vi "EINDE2.vi"() -> ()   [LabVIEW 2018]
uses:
  Kleuren- en afstandsensor/FSM States.ctl
  FSM States Project TOTAAL.ctl
panel:
  out "Initial State":T1=enum."MOVE DOWNWARDS"
  out "Tussentijd":i32
  out "Timer":i32
  out "The End":bool
  in  "stop 3":bool
  in  "ON/OFF Grijper":bool
  in  "stop":bool
  in  "Aantal Witte blokjes":dbl
  in  "Aantal rode blokjes":dbl
  in  "Aantal Zwarte blokjes":dbl
  in  "LED aansturen":bool[](array[boolean])
  out "Current State":T1
  out "Motor":bool[](array[boolean])
  out "State to recover from":T1=enum."Stilstaan"
  in  "EMERGENCY":bool
  in  "Teller wit":dbl
  in  "Teller Rood":dbl
  in  "Teller zwart":dbl
  out "Wit":bool
  out "Zwart":bool
  out "Rood":bool
  in  "Kleurmaken":bool
  out "Kleuren veranderen":T2
  out "Analoge in":dbl[](array[numeric]) format="%0.2f"
  out "Afstand":bool
  # "INPUT"
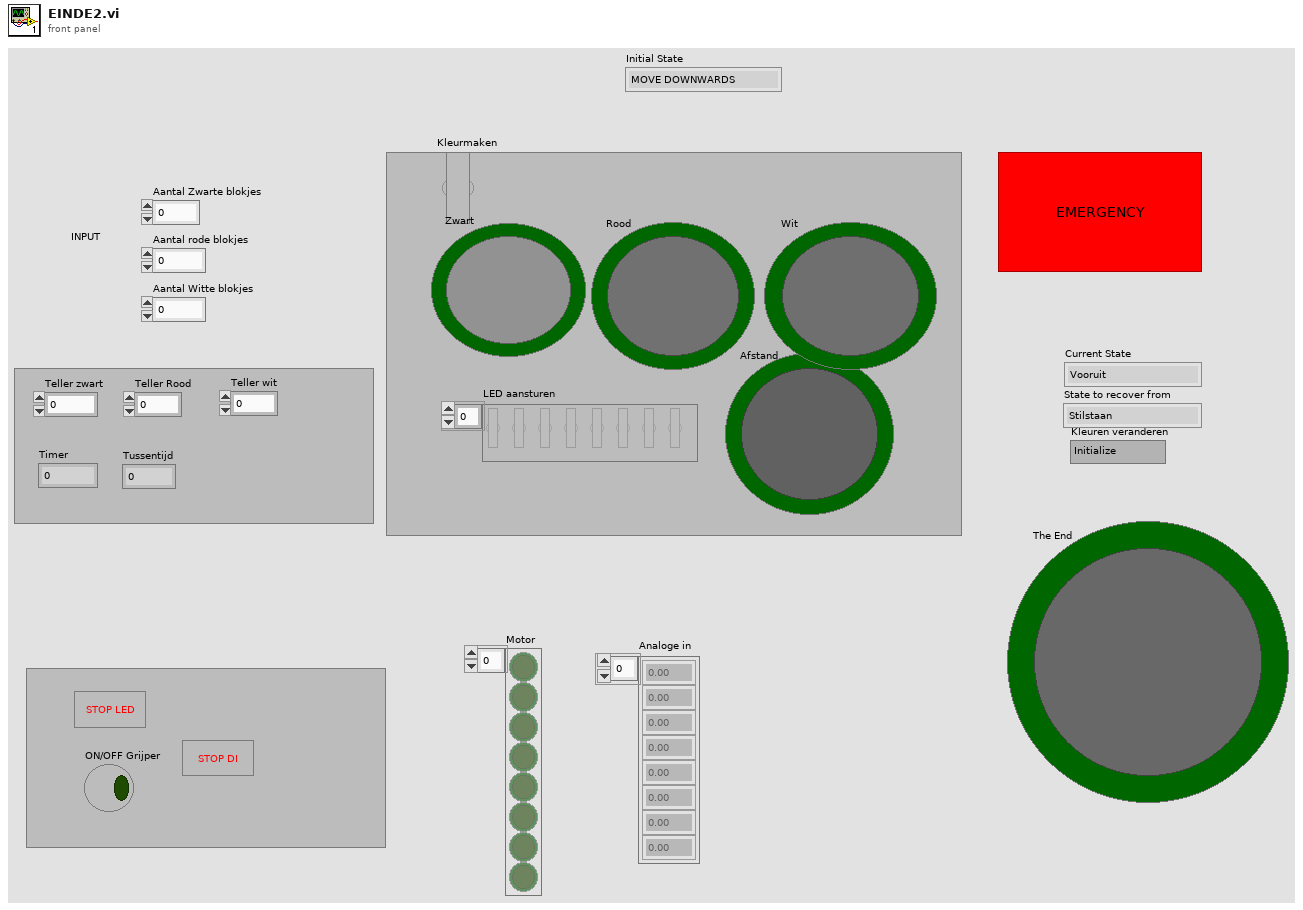
[diagram p1: front panel]
types:
  T1 = typedef "FSM States Project TOTAAL.ctl" = enum16{"Vooruit", "Achteruit", "Stilstaan", "EMERGENCY", "MOVE DOWNWARDS", "GRAB", "MOVE UPWARDS", "ROTATE", "DROP", "RETURN", "Stop "}
  T2 = typedef "FSM States.ctl" = enum16{"Initialize", "ROOD", "GROEN ", "Blauw "}
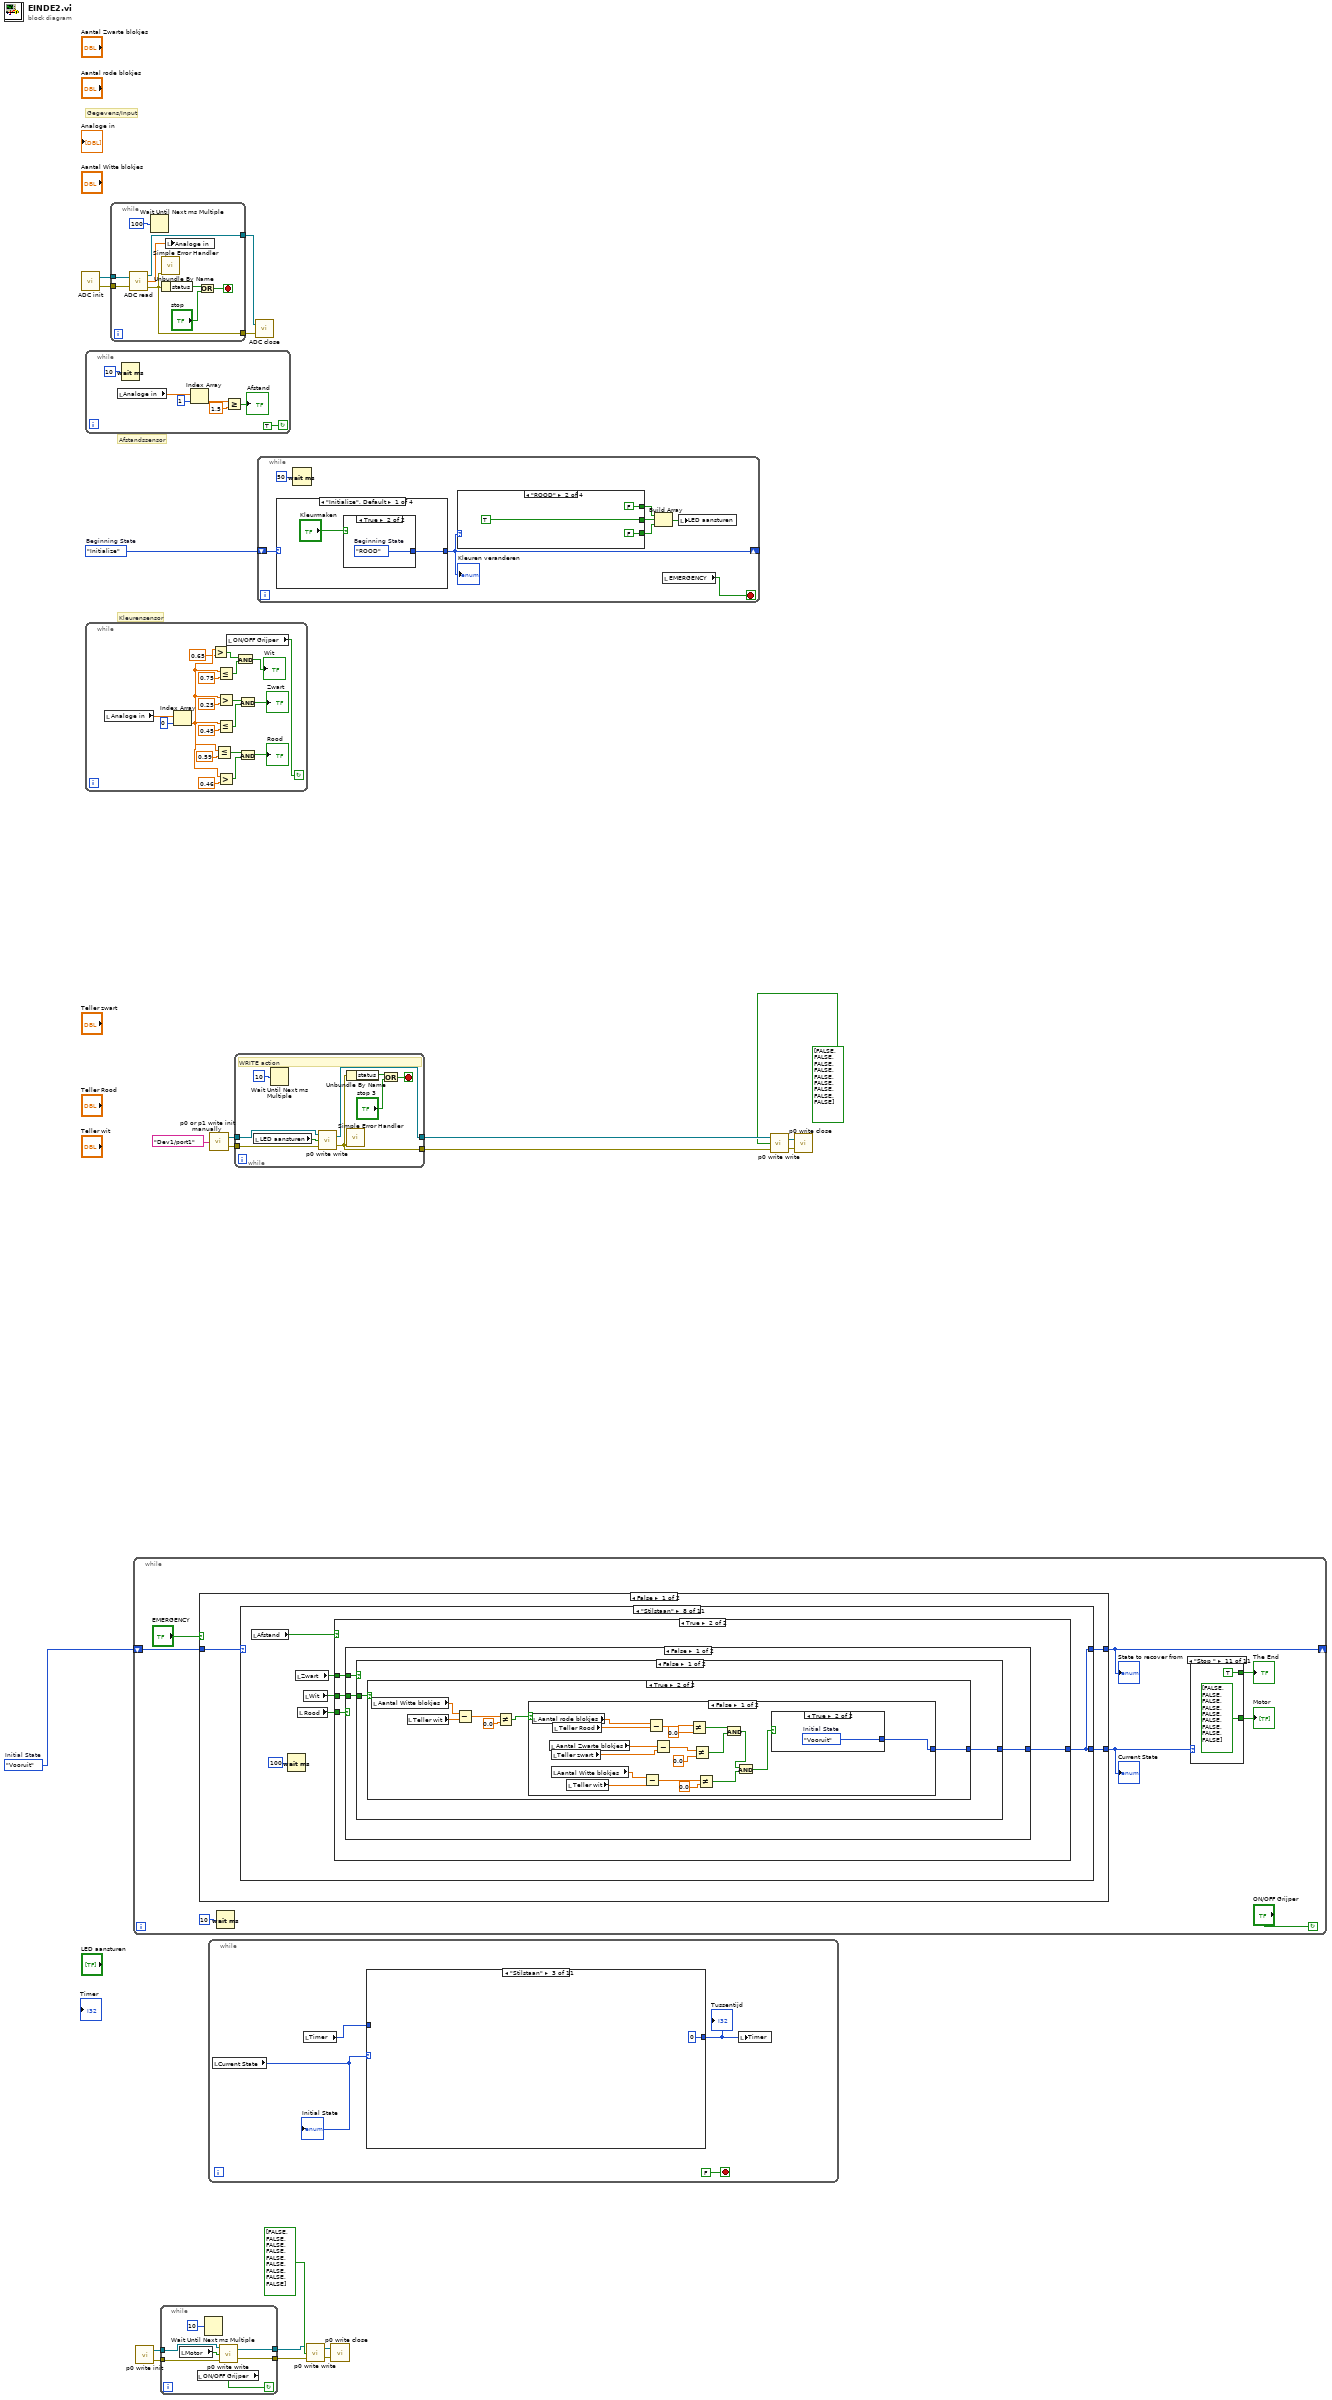
[diagram p0: block diagram]
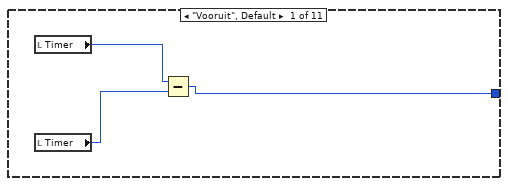
[diagram p2: hidden frame]
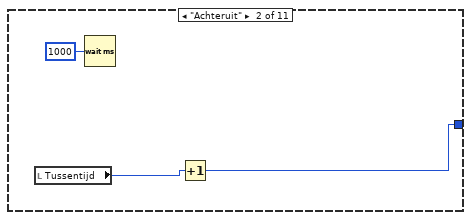
[diagram p3: hidden frame]
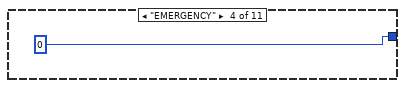
[diagram p4: hidden frame]
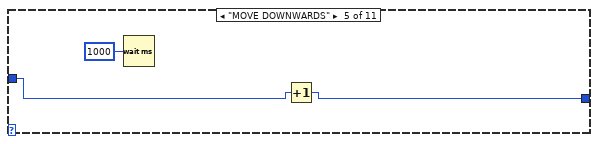
[diagram p5: hidden frame]
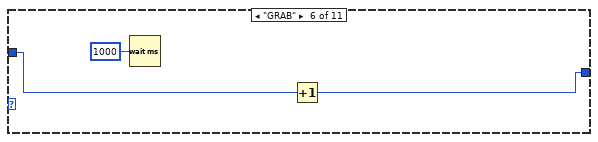
[diagram p6: hidden frame]
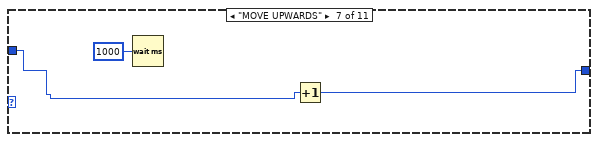
[diagram p7: hidden frame]
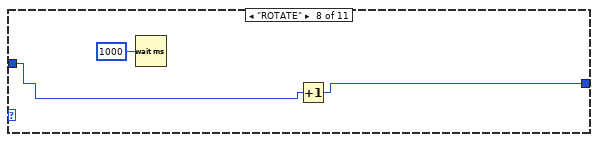
[diagram p8: hidden frame]
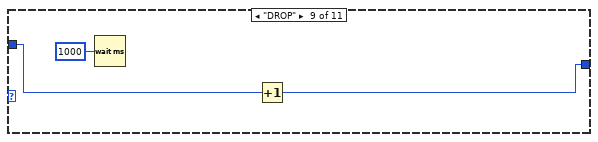
[diagram p9: hidden frame]
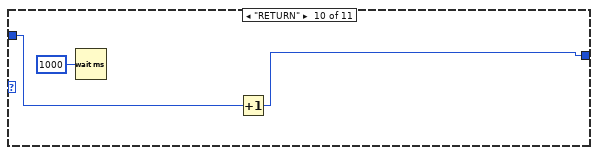
[diagram p10: hidden frame]
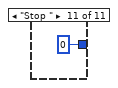
[diagram p11: hidden frame]
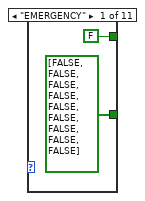
[diagram p12: hidden frame]
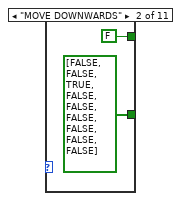
[diagram p13: hidden frame]
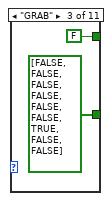
[diagram p14: hidden frame]
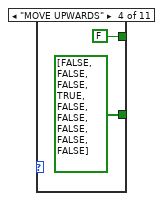
[diagram p15: hidden frame]
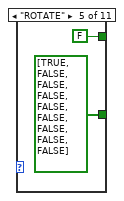
[diagram p16: hidden frame]
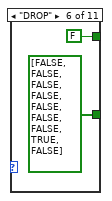
[diagram p17: hidden frame]
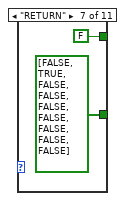
[diagram p18: hidden frame]
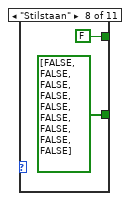
[diagram p19: hidden frame]
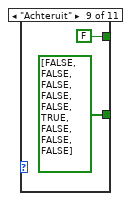
[diagram p20: hidden frame]
diagram:
  w1 = FSM_States_Project_TOTAAL."Vooruit"  # Initial State
  w17 = FSM_States."Initialize"  # Beginning State
  # "Gegevens/Input"
  # "Kleurensensor"
  # "Afstandssensor"
  n1 = call "ADC init.vi"() -> ("error out"=w20:errorcluster, "task out"=w21:refnum<k21>)
  n2 = while {
    stop <- TRUE continue-if-true
    n3 = local read "Analoge in"() -> (w22:dbl[])
    n4 = Wait (ms)(milliseconds to wait=u32 10) -> ()  [unwired: 1 out]
    n5 = Index Array(array=w22, index=1) -> (element=w26:dbl)
    n6 = Greater Or Equal?(x=w26, y=1.5) -> (x >= y?=→"Afstand":bool)
  }
  n7 = while {
    stop <- w34 continue-if-true
    n8 = local read "Analoge in"() -> (w46:dbl[])
    n9 = Index Array(array=w46, index=0) -> (element=w30:dbl)
    n10 = Greater?(x=w30, y=0.65) -> (0:w31:bool)
    n11 = Less Or Equal?(x=w30, y=0.59) -> (x <= y?=w36:bool)
    n12 = Less Or Equal?(x=w30, y=0.75) -> (x <= y?=w33:bool)
    n13 = Greater?(x=w30, y=0.25) -> (0:w42:bool)
    n14 = Less Or Equal?(x=w30, y=0.45) -> (x <= y?=w41:bool)
    n15 = Greater?(x=w30, y=0.46) -> (0:w35:bool)
    n16 = local read "ON/OFF Grijper"() -> (w34:bool)
    n17 = And(x=w31, y=w33) -> (x .and. y?=→"Wit":bool)
    n18 = And(x=w42, y=w41) -> (x .and. y?=→"Zwart":bool)
    n19 = And(x=w36, y=w35) -> (x .and. y?=→"Rood":bool)
  }
  n20 = while {
    tunnel: w21 -> [w56]
    tunnel: w20 -> [w55]
    tunnel: [w52] -> w19
    tunnel: [w54] -> w18
    stop <- w49 stop-if-true
    n21 = call "ADC read.vi"("task/channels in"=w56, "error in"=w55) -> ("task out"=w54:refnum<k21>, "analog in"=w48:dbl[], "error out"=w52:errorcluster)
    n22 = Wait Until Next ms Multiple(millisecond multiple=u32 100) -> ()  [unwired: 1 out]
    n23 = call <vilib>:"Simple Error Handler.vi"("error in (no error)"=w52) -> ()  [unwired: 4 in, 5 out]
    n24 = Unbundle By Name(w52) -> ("status"=w51:bool)
    n25 = local write "Analoge in"(w48) -> ()
    n26 = Or(x=w51, y="stop") -> (x .or. y?=w49:bool)
  }
  n27 = while {
    shift-right: [w60] -> _
    shift-left: w1 -> [w61]
    stop <- "ON/OFF Grijper" continue-if-true
    n28 = case shown="False" "EMERGENCY" {
      tunnel: w61 -> [w89 _]
      tunnel: [w88 FSM_States_Project_TOTAAL."EMERGENCY" ("State to Recover from 2")] -> w59
      tunnel: [w87 w204] -> w60
      frame False {
        n29 = case shown="\"Stilstaan\"" w89 {
          tunnel: [w90 w91 w97 w103 w109 w115 w121 w132 w196 w199 w203] -> w88
          tunnel: [w90 w91 w97 w103 w109 w115 w121 w132 w196 w199 w203] -> w87
          frame "EMERGENCY" {
            n30 = local read "State to recover from"() -> (w90:T1)
          }
          frame "MOVE DOWNWARDS" {
            n31 = local read "Timer"() -> (w94:i32)
            n32 = Greater Or Equal?(x=w94, y=8) -> (x >= y?=w92:bool)
            n33 = case shown="False" w92 {
              tunnel: [FSM_States_Project_TOTAAL."MOVE DOWNWARDS" FSM_States_Project_TOTAAL."GRAB"] -> w91
              frame False {
              }
              frame True {
              }
            }
          }
          frame "GRAB" {
            n34 = local read "Timer"() -> (w99:i32)
            n35 = Greater Or Equal?(x=w99, y=10) -> (x >= y?=w100:bool)
            n36 = case shown="True" w100 {
              tunnel: [w101 w102] -> w97
              frame False {
                w101 = FSM_States_Project_TOTAAL."GRAB"  # Next State
              }
              frame True {
                w102 = FSM_States_Project_TOTAAL."MOVE UPWARDS"  # Next State
              }
            }
          }
          frame "MOVE UPWARDS" {
            n37 = local read "Timer"() -> (w106:i32)
            n38 = Greater Or Equal?(x=w106, y=20) -> (x >= y?=w104:bool)
            n39 = case shown="True" w104 {
              tunnel: [w107 w108] -> w103
              frame False {
                w107 = FSM_States_Project_TOTAAL."MOVE UPWARDS"  # Next State
              }
              frame True {
                w108 = FSM_States_Project_TOTAAL."ROTATE"  # Next State
              }
            }
          }
          frame "ROTATE" {
            n40 = local read "Timer"() -> (w112:i32)
            n41 = Greater Or Equal?(x=w112, y=23) -> (x >= y?=w110:bool)
            n42 = case shown="False" w110 {
              tunnel: [w113 w114] -> w109
              frame False {
                w113 = FSM_States_Project_TOTAAL."ROTATE"  # Next State
              }
              frame True {
                w114 = FSM_States_Project_TOTAAL."DROP"  # Next State
              }
            }
          }
          frame "DROP" {
            n43 = local read "Timer"() -> (w118:i32)
            n44 = Greater Or Equal?(x=w118, y=25) -> (x >= y?=w116:bool)
            n45 = case shown="True" w116 {
              tunnel: [w119 w120] -> w115
              frame False {
                w119 = FSM_States_Project_TOTAAL."DROP"  # Next State
              }
              frame True {
                w120 = FSM_States_Project_TOTAAL."RETURN"  # Next State
              }
            }
          }
          frame "RETURN" {
            n46 = local read "Timer"() -> (w123:i32)
            n47 = Greater Or Equal?(x=w123, y=28) -> (x >= y?=w124:bool)
            n48 = case shown="True" w124 {
              tunnel: [w125 w126] -> w121
              frame False {
                w125 = FSM_States_Project_TOTAAL."RETURN"  # Next State
              }
              frame True {
                w126 = FSM_States_Project_TOTAAL."Vooruit"  # Next State
              }
            }
          }
          frame "Stilstaan" {
            n49 = local read "Afstand"() -> (w131:bool)
            n50 = Wait (ms)(milliseconds to wait=u32 100) -> ()  [unwired: 1 out]
            n51 = local read "Zwart"() -> (w129:bool)
            n52 = local read "Rood"() -> (w130:bool)
            n53 = local read "Wit"() -> (w128:bool)
            n54 = case shown="True" w131 {
              tunnel: [w133 w137] -> w132
              tunnel: w130 -> [_ w136]
              tunnel: w129 -> [_ w135]
              tunnel: w128 -> [_ w134]
              frame False {
                w133 = FSM_States_Project_TOTAAL."Vooruit"  # Initial State
              }
              frame True {
                n55 = case shown="False" w136 {
                  tunnel: [w140 w188] -> w137
                  tunnel: w135 -> [w139 _]
                  tunnel: w134 -> [w138 _]
                  frame False {
                    n56 = case shown="False" w139 {
                      tunnel: [w142 w178] -> w140
                      tunnel: w138 -> [w141 _]
                      frame False {
                        n57 = case shown="True" w141 {
                          tunnel: [w143 w149] -> w142
                          frame False {
                            w143 = FSM_States_Project_TOTAAL."Stilstaan"  # Initial State
                          }
                          frame True {
                            n58 = local read "Aantal Witte blokjes"() -> (w146:dbl)
                            n59 = local read "Teller wit"() -> (w147:dbl)
                            n60 = Subtract(x=w146, y=w147) -> (x-y=w148:dbl)
                            n61 = Not Equal?(x=w148, y=0.0) -> (x != y?=w144:bool)
                            n62 = case shown="False" w144 {
                              tunnel: [w150 w170] -> w149
                              frame False {
                                n63 = local read "Aantal rode blokjes"() -> (w167:dbl)
                                n64 = local read "Aantal Zwarte blokjes"() -> (w163:dbl)
                                n65 = local read "Teller zwart"() -> (w162:dbl)
                                n66 = local read "Aantal Witte blokjes"() -> (w158:dbl)
                                n67 = local read "Teller Rood"() -> (w166:dbl)
                                n68 = local read "Teller wit"() -> (w157:dbl)
                                n69 = Subtract(x=w158, y=w157) -> (x-y=w156:dbl)
                                n70 = Subtract(x=w167, y=w166) -> (x-y=w165:dbl)
                                n71 = Subtract(x=w163, y=w162) -> (x-y=w161:dbl)
                                n72 = Not Equal?(x=w165, y=0.0) -> (x != y?=w155:bool)
                                n73 = Not Equal?(x=w161, y=0.0) -> (x != y?=w154:bool)
                                n74 = Not Equal?(x=w156, y=0.0) -> (x != y?=w153:bool)
                                n75 = And(x=w155, y=w154) -> (x .and. y?=w152:bool)
                                n76 = And(x=w152, y=w153) -> (x .and. y?=w151:bool)
                                n77 = case shown="True" w151 {
                                tunnel: [w168 w169] -> w150
                                frame False {
                                w168 = FSM_States_Project_TOTAAL."Achteruit"  # Initial State
                                }
                                frame True {
                                w169 = FSM_States_Project_TOTAAL."Vooruit"  # Initial State
                                }
                                }
                              }
                              frame True {
                                w170 = FSM_States_Project_TOTAAL."MOVE DOWNWARDS"  # Initial State
                                n78 = local read "Teller wit"() -> (w172:dbl)
                                n79 = Increment(x=w172) -> (x+1=w171:dbl)
                                n80 = local write "Teller wit"(w171) -> ()
                              }
                            }
                          }
                        }
                      }
                      frame True {
                        n81 = local read "Aantal Zwarte blokjes"() -> (w176:dbl)
                        n82 = local read "Teller zwart"() -> (w177:dbl)
                        n83 = Subtract(x=w176, y=w177) -> (x-y=w174:dbl)
                        n84 = Not Equal?(x=w174, y=0.0) -> (x != y?=w173:bool)
                        n85 = case shown="False" w173 {
                          tunnel: [w179 w180] -> w178
                          frame False {
                            w179 = FSM_States_Project_TOTAAL."Vooruit"  # Initial State
                          }
                          frame True {
                            w180 = FSM_States_Project_TOTAAL."MOVE DOWNWARDS"  # Initial State
                            n86 = local read "Teller zwart"() -> (w182:dbl)
                            n87 = Increment(x=w182) -> (x+1=w181:dbl)
                            n88 = local write "Teller zwart"(w181) -> ()
                          }
                        }
                      }
                    }
                  }
                  frame True {
                    n89 = local read "Aantal rode blokjes"() -> (w187:dbl)
                    n90 = local read "Teller Rood"() -> (w186:dbl)
                    n91 = Subtract(x=w187, y=w186) -> (x-y=w184:dbl)
                    n92 = Not Equal?(x=w184, y=0.0) -> (x != y?=w183:bool)
                    n93 = case shown="False" w183 {
                      tunnel: [w189 w192] -> w188
                      frame False {
                        w189 = FSM_States_Project_TOTAAL."Vooruit"  # Initial State
                      }
                      frame True {
                        w192 = FSM_States_Project_TOTAAL."MOVE DOWNWARDS"  # Initial State
                        n94 = local read "Teller Rood"() -> (w191:dbl)
                        n95 = Increment(x=w191) -> (x+1=w190:dbl)
                        n96 = local write "Teller Rood"(w190) -> ()
                      }
                    }
                  }
                }
              }
            }
          }
          frame "Achteruit" {
            n97 = local read "Tussentijd"() -> (w195:i32)
            n98 = Equal?(x=w195, y=5) -> (x = y?=w193:bool)
            n99 = case shown="True" w193 {
              tunnel: [w197 w198] -> w196
              frame False {
                w197 = FSM_States_Project_TOTAAL."Achteruit"  # Initial State
              }
              frame True {
                w198 = FSM_States_Project_TOTAAL."Stop "  # Initial State
              }
            }
          }
          frame "Vooruit" {
            n100 = local read "Afstand"() -> (w200:bool)
            n101 = case shown="False" w200 {
              tunnel: [w201 w202] -> w199
              frame False {
                w201 = FSM_States_Project_TOTAAL."Vooruit"  # Initial State
              }
              frame True {
                w202 = FSM_States_Project_TOTAAL."Stilstaan"  # Initial State
              }
            }
          }
          frame "Stop " {
            w203 = FSM_States_Project_TOTAAL."Stop "  # Initial State
          }
        }
      }
      frame True {
        n102 = local read "State to recover from"() -> (w204:T1)
      }
    }
    "State to recover from" <- w60
    "Current State" <- w59
    n103 = Wait (ms)(milliseconds to wait=u32 10) -> ()  [unwired: 1 out]
    n104 = case shown="\"Stop \"" w59 {
      tunnel: [bool[] [FALSE, FALSE, FALSE, FALSE, FALSE, FALSE, FALSE, FALSE, FALSE] ("digital out") bool[] [FALSE, FALSE, TRUE, FALSE, FALSE, FALSE, FALSE, FALSE, FALSE] ("digital out") bool[] [FALSE, FALSE, FALSE, FALSE, FALSE, FALSE, TRUE, FALSE, FALSE] ("digital out") bool[] [FALSE, FALSE, FALSE, TRUE, FALSE, FALSE, FALSE, FALSE, FALSE] ("digital out") bool[] [TRUE, FALSE, FALSE, FALSE, FALSE, FALSE, FALSE, FALSE, FALSE] ("digital out") bool[] [FALSE, FALSE, FALSE, FALSE, FALSE, FALSE, FALSE, TRUE, FALSE] ("digital out") bool[] [FALSE, TRUE, FALSE, FALSE, FALSE, FALSE, FALSE, FALSE, FALSE] ("digital out") bool[] [FALSE, FALSE, FALSE, FALSE, FALSE, FALSE, FALSE, FALSE, FALSE] ("digital out") bool[] [FALSE, FALSE, FALSE, FALSE, FALSE, TRUE, FALSE, FALSE, FALSE] ("digital out") bool[] [FALSE, FALSE, FALSE, FALSE, TRUE, FALSE, FALSE, FALSE, FALSE] ("digital out") bool[] [FALSE, FALSE, FALSE, FALSE, FALSE, FALSE, FALSE, FALSE, FALSE] ("digital out")] -> w57
      tunnel: [FALSE ("The End") FALSE ("The End") FALSE ("The End") FALSE ("The End") FALSE ("The End") FALSE ("The End") FALSE ("The End") FALSE ("The End") FALSE ("The End") FALSE ("The End") TRUE ("The End")] -> w58
      frame "EMERGENCY" {
      }
      frame "MOVE DOWNWARDS" {
      }
      frame "GRAB" {
      }
      frame "MOVE UPWARDS" {
      }
      frame "ROTATE" {
      }
      frame "DROP" {
      }
      frame "RETURN" {
      }
      frame "Stilstaan" {
      }
      frame "Achteruit" {
      }
      frame "Vooruit" {
      }
      frame "Stop " {
      }
    }
    "Motor" <- w57
    "The End" <- w58
  }
  n105 = call "p0 write init.vi"() -> ("error out"=w3:errorcluster, "task out"=w2:refnum<k21>)
  n106 = while {
    tunnel: [w211] -> w5
    tunnel: [w210] -> w4
    tunnel: w3 -> [w208]
    tunnel: w2 -> [w209]
    stop <- w212 continue-if-true
    n107 = local read "Motor"() -> (w206:bool[])
    n108 = local read "ON/OFF Grijper"() -> (w212:bool)
    n109 = Wait Until Next ms Multiple(millisecond multiple=u32 10) -> ()  [unwired: 1 out]
    n110 = call "p0 write write.vi"("error in"=w208, "digital out"=w206, "task/channels in"=w209) -> ("error out"=w211:errorcluster, "task out"=w210:refnum<k21>)
  }
  n111 = while {
    stop <- FALSE stop-if-true
    n112 = local read "Current State"() -> (w213:T1)
    "Initial State" <- w213
    n113 = local read "Timer"() -> (w215:i32)
    n114 = case shown="\"Stilstaan\"" w213 {
      tunnel: w215 -> [_ _ _ _ w226 w229 w232 w235 w238 w241 _]
      tunnel: [w219 w220 0 ("Timer2") 0 ("Timer2") w225 w228 w231 w234 w237 w240 0 ("Timer2")] -> w214
      frame "Vooruit", Default {
        n115 = local read "Timer"() -> (w217:i32)
        n116 = local read "Timer"() -> (w218:i32)
        n117 = Subtract(x=w217, y=w218) -> (x-y=w219:i32)
      }
      frame "Achteruit" {
        n118 = local read "Tussentijd"() -> (w221:i32)
        n119 = Wait (ms)(milliseconds to wait=u32 1000) -> ()  [unwired: 1 out]
        n120 = Increment(x=w221) -> (x+1=w220:i32)
      }
      frame "Stilstaan" {
      }
      frame "EMERGENCY" {
      }
      frame "MOVE DOWNWARDS" {
        n121 = Wait (ms)(milliseconds to wait=u32 1000) -> ()  [unwired: 1 out]
        n122 = Increment(x=w226) -> (x+1=w225:i32)
      }
      frame "GRAB" {
        n123 = Wait (ms)(milliseconds to wait=u32 1000) -> ()  [unwired: 1 out]
        n124 = Increment(x=w229) -> (x+1=w228:i32)
      }
      frame "MOVE UPWARDS" {
        n125 = Wait (ms)(milliseconds to wait=u32 1000) -> ()  [unwired: 1 out]
        n126 = Increment(x=w232) -> (x+1=w231:i32)
      }
      frame "ROTATE" {
        n127 = Wait (ms)(milliseconds to wait=u32 1000) -> ()  [unwired: 1 out]
        n128 = Increment(x=w235) -> (x+1=w234:i32)
      }
      frame "DROP" {
        n129 = Wait (ms)(milliseconds to wait=u32 1000) -> ()  [unwired: 1 out]
        n130 = Increment(x=w238) -> (x+1=w237:i32)
      }
      frame "RETURN" {
        n131 = Wait (ms)(milliseconds to wait=u32 1000) -> ()  [unwired: 1 out]
        n132 = Increment(x=w241) -> (x+1=w240:i32)
      }
      frame "Stop " {
      }
    }
    "Tussentijd" <- w214
    n133 = local write "Timer"(w214) -> ()
  }
  n134 = call "p0 or p1 write init manually.vi"("Port"=tag "Dev1/port1") -> ("task out"=w11:refnum<k21>, "error out"=w10:errorcluster)
  n135 = while {
    tunnel: w11 -> [w252]
    tunnel: [w251] -> w16
    tunnel: w10 -> [w250]
    tunnel: [w246] -> w15
    stop <- w247 stop-if-true
    # "WRITE action"
    n136 = local read "LED aansturen"() -> (w244:bool[])
    n137 = Wait Until Next ms Multiple(millisecond multiple=u32 10) -> ()  [unwired: 1 out]
    n138 = call "p0 write write.vi"("error in"=w250, "digital out"=w244, "task/channels in"=w252) -> ("error out"=w246:errorcluster, "task out"=w251:refnum<k21>)
    n139 = Unbundle By Name(w246) -> ("status"=w245:bool)
    n140 = call <vilib>:"Simple Error Handler.vi"("error in (no error)"=w246) -> ()  [unwired: 4 in, 5 out]
    n141 = Or(x=w245, y="stop 3") -> (x .or. y?=w247:bool)
  }
  n142 = call "ADC close.vi"("error in"=w19, "task/channels in"=w18) -> ()
  n143 = while {
    shift-right: [w254] -> _
    shift-left: w17 -> [w260]
    stop <- w253 stop-if-true
    n144 = case shown="\"Initialize\", Default" w260 {
      tunnel: [w274 w277 w278 w279] -> w254
      frame "Initialize", Default {
        n145 = case shown="True" "Kleurmaken" {
          tunnel: [w275 w276] -> w274
          frame False {
            w275 = FSM_States."Initialize"  # Beginning State
          }
          frame True {
            w276 = FSM_States."ROOD"  # Beginning State
          }
        }
      }
      frame "ROOD" {
        w277 = FSM_States."GROEN "  # Beginning State
      }
      frame "GROEN " {
        w278 = FSM_States."Blauw "  # Beginning State
      }
      frame "Blauw " {
        w279 = FSM_States."ROOD"  # Beginning State
      }
    }
    "Kleuren veranderen" <- w254
    n146 = Wait (ms)(milliseconds to wait=u32 50) -> ()  [unwired: 1 out]
    n147 = case shown="\"ROOD\"" w254 {
      tunnel: [FALSE FALSE FALSE TRUE] -> w257
      tunnel: [FALSE TRUE FALSE FALSE] -> w256
      tunnel: [FALSE FALSE TRUE FALSE] -> w255
      frame "Initialize", Default {
      }
      frame "ROOD" {
      }
      frame "GROEN " {
      }
      frame "Blauw " {
      }
    }
    n148 = Build Array(w257, w256, w255) -> (w258:bool[])
    n149 = local read "EMERGENCY"() -> (w253:bool)
    n150 = local write "LED aansturen"(w258) -> ()
  }
  n151 = call "p0 write write.vi"("error in"=w5, "digital out"=bool[] [FALSE, FALSE, FALSE, FALSE, FALSE, FALSE, FALSE, FALSE, FALSE], "task/channels in"=w4) -> ("error out"=w7:errorcluster, "task out"=w8:refnum<k21>)
  n152 = call "p0 write close.vi"("error in"=w7, "task/channels in"=w8) -> ()
  n153 = call "p0 write write.vi"("error in"=w15, "digital out"=bool[] [FALSE, FALSE, FALSE, FALSE, FALSE, FALSE, FALSE, FALSE, FALSE], "task/channels in"=w16) -> ("error out"=w13:errorcluster, "task out"=w14:refnum<k21>)
  n154 = call "p0 write close.vi"("error in"=w13, "task/channels in"=w14) -> ()
